vi "Setup Statically-Linked subWorkers.vi"(8 "error in":errorcluster, 11 "DAQ Worker in":refnum<class "DAQ Worker.lvclass">) -> (0 "error out":errorcluster, 3 "DAQ Worker out":refnum<class "DAQ Worker.lvclass">)   [LabVIEW 2020, in "DAQ Worker.lvclass"]
doc: "This VI performs a setup of all the statically-linked subWorkers that belong to the Worker that owns this VI. This VI must be called <b>before</b> any statically-linked subWorkers are called."
uses:
  DAQ Worker.lvclass
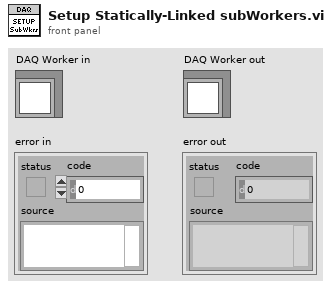
[diagram p1: front panel]
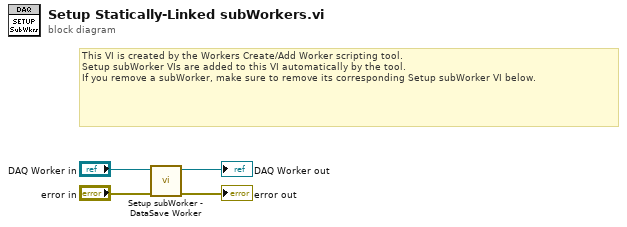
[diagram p0: block diagram]
diagram:
  # "This VI is created by the Workers Create/Add Worker scripting tool.\nSetup subWorker VIs are added to this VI automatically by the tool.\nIf you remove a subWorker, make sure to remove its corresponding Setup subWorker VI below."
  n1 = call "Setup subWorker - DataSave Worker.vi"("error in"="error in", "DAQ Worker in"="DAQ Worker in") -> ("error out"=→"error out":errorcluster, "DAQ Worker out"=→"DAQ Worker out":refnum<class "DAQ Worker.lvclass">)  [unwired: 8 in]
